vi "Mother Wavelet and Scaling Function.vi"() -> ()   [LabVIEW 2023]
doc: "This example shows how to estimate the mother wavelet function and the scaling function from the wavelet filter coefficients with the WA Mother Wavelet and Scaling Function VI. When <B>Refinement</B> increases, the estimated mother wavelet function and scaling function precisely approximate to the real values.\n\n<b>Instructions:</b>\n1) Run this VI.\n2) Observe the <b>Lowpass Filter</b>, <b>Highpass Filter</b>, <b>Scaling Function</b> and <b>Mother Wavelet Function</b> by using different <b>Wavelet</b> types."
uses:
  <vilib>/addons/_Advanced Signal Processing/NI_AdvSigProcWA.lvlib
panel:
  out "aspt-left-top":bool
  in  "stop":bool
  in  "Refinement":i32=5 min=1 max=10 step=1
  out "Mother Wavelet Function":T1(graph)
  out "Scaling Function":T2(graph)
  out "Highpass Filter":dbl[](graph)
  out "Lowpass Filter":dbl[](graph)
  in  "Wavelet":u16(ring) items=["db02"=0, "db03"=1, "db04"=2, "db05"=3, "db06"=4, "db07"=5, "db08"=6, "db09"=7, "db10"=8, "db11"=9, "db12"=10, "db13"=11, "db14"=12, "Haar"=13, "bior1_3"=14, "bior1_5"=15, "bior2_2"=16, "bior2_4"=17, "bior2_6"=18, "bior2_8"=19, "bior3_1"=20, "bior3_3"=21, "bior3_5"=22, "bior3_7"=23, "bior3_9"=24, "bior4_4 (FBI)"=25, "bior5_5"=38, "bior6_8"=39, "coif1"=26, "coif2"=27, "coif3"=28, "coif4"=29, "coif5"=30, "sym2"=31, "sym3"=32, "sym4"=33, "sym5"=34, "sym6"=35, "sym7"=36, "sym8"=37]
  # "Overview: Shows how to estimate the mother wavelet function and the scaling function from the wavelet filter coefficients with the WA Mother Wavelet and Scaling Function VI. \nRequirements: LabVIEW Full Development System, Advanced Signal Processing Toolkit\nInstructions: \n1. Run this VI.\n2. Observe the Lowpass Filter, Highpass Filter, Scaling Function and Mother Wavelet Function by using different Wavelet types.\n3. Click Stop to stop the VI."
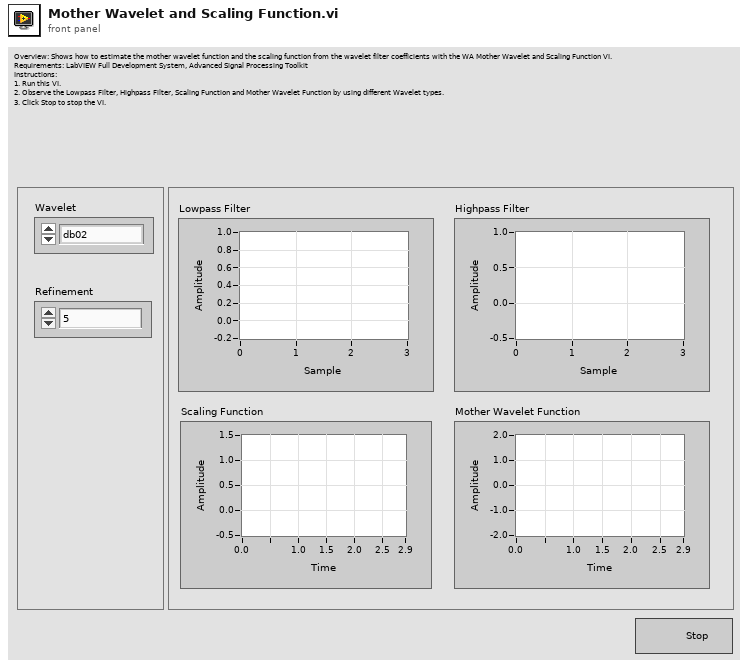
[diagram p1: front panel]
types:
  T1 = cluster{"t0":dbl, "dt":dbl, "wavelet function":dbl[]}
  T2 = cluster{"t0":dbl, "dt":dbl, "scaling function":dbl[]}
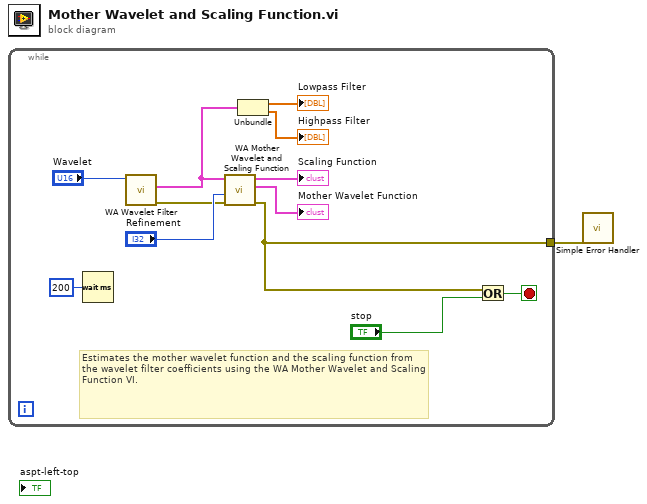
[diagram p0: block diagram]
diagram:
  n1 = while {
    tunnel: [w2] -> w1
    stop <- w5 stop-if-true
    # "Estimates the mother wavelet function and the scaling function from the wavelet filter coefficients using the WA Mother Wavelet and Scaling Function VI."
    n2 = Wait (ms)(milliseconds to wait=u32 200 ("millisecond multiple")) -> ()  [unwired: 1 out]
    n3 = call <vilib>:"WA Wavelet Filter.vi"("wavelet"="Wavelet") -> ("error out"=w3:errorcluster, "analysis filters"=w12:cluster{"lowpass":dbl[], "highpass":dbl[]})  [unwired: 3 in, 6 out]
    n4 = call <vilib>:"WA Mother Wavelet and Scaling Function.vi"("error in (no error)"=w3, "refinements"="Refinement", "filters"=w12) -> ("error out"=w2:errorcluster, "mother wavelet function info"=→"Mother Wavelet Function":T1, "scaling function info"=→"Scaling Function":T2)  [unwired: 6 out]
    n5 = Unbundle(w12) -> ("lowpass"=→"Lowpass Filter":dbl[], "highpass"=→"Highpass Filter":dbl[])
    n6 = Or(x=w2, y="stop") -> (x .or. y?=w5:bool)
  }
  n7 = call <vilib>:"Simple Error Handler.vi"("error in (no error)"=w1) -> ()  [unwired: 1 in, 8 out]
